vi "Load or Save OM Location.vi"(2 "error in (no error)":errorcluster, 3 "Action":T2=enum."Load") -> (0 "error out":errorcluster, 1 "LBCB  Location Out":T1)   [LabVIEW 2009]
uses:
  Data Access Objects/Metadata/Persistant DAO Actions.ctl
  Data Access Objects/Metadata/LBCB Location.ctl
  ConfigPathActions.ctl
  <vilib>/Utility/config.llb/NI_LVConfig.lvlib
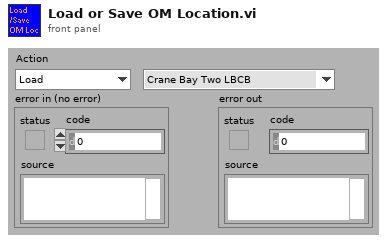
[diagram p1: front panel]
types:
  T1 = typedef "LBCB Location.ctl" = enum16{"Crane Bay Two LBCB", "Crane Bay One LBCB", "5th Scale Two LBCB", "5th Scale One LBCB", "Portable LBCB"}
  T2 = typedef "Persistant DAO Actions.ctl" = enum16{"Init", "Get", "Set", "Load", "Save"}
  T3 = typedef "ConfigPathActions.ctl" = enum16{"Init", "Application", "MixedMode", "ControlLoop", "Calibration", "System", "Change Location"}
  T4 = typedef "NI_LVConfig.lvlib/Config Data RefNum.ctl" = refnum<k1>
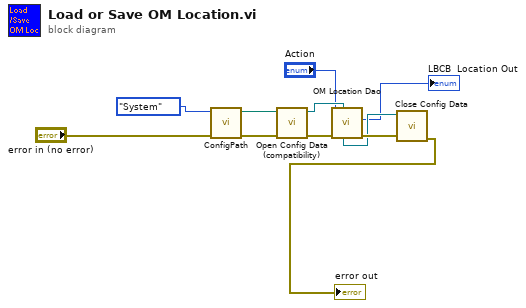
[diagram p0: block diagram]
diagram:
  n1 = call "ConfigPath.vi"("error in (no error)"="error in (no error)", "Config Path Actions"=ConfigPathActions."System") -> ("error out"=w2:errorcluster, "Path"=w3:path)  [unwired: 1 in, 7 out]
  n2 = call <vilib>:"Open Config Data (compatibility).vi"("error in (no error)"=w2, "configuration file path"=w3) -> ("error out"=w10:errorcluster, "refnum"=w5:T4)  [unwired: 7 in, 1 out]
  n3 = call "OM Location Dao.vi"("Config Ref Number"=w5, "error in (no error)"=w10, "Actions"="Action") -> ("error out"=w7:errorcluster, "LBCB  Location Out"=→"LBCB  Location Out":T1, "Config Ref Number out"=w6:T4)  [unwired: 1 in, 5 out]
  n4 = call <vilib>:"Close Config Data.vi"("error in (no error)"=w7, "refnum"=w6) -> ("error out"=→"error out":errorcluster)  [unwired: 1 in, 8 out]
